vi "picoharp_close_device_handle.vi"(8 "error in (no error)":errorcluster, 11 "hydraharp in":refnum<class "picoharp.lvclass">) -> (0 "error out":errorcluster, 3 "hydraharp out":refnum<class "picoharp.lvclass">)   [LabVIEW 2015, in "picoharp.lvclass"]
uses:
  picoharp.lvclass
  picoharp.lvclass/picoharp.ctl
  phlib.dll
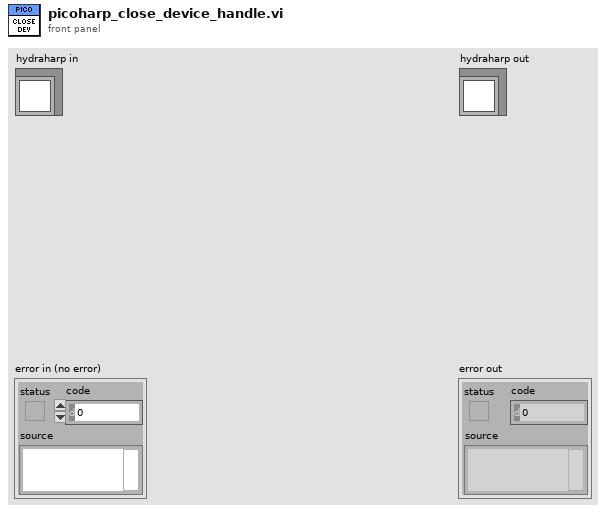
[diagram p1: front panel]
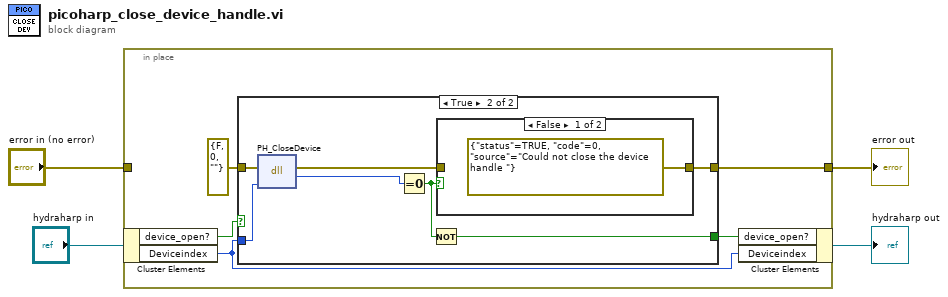
[diagram p0: block diagram]
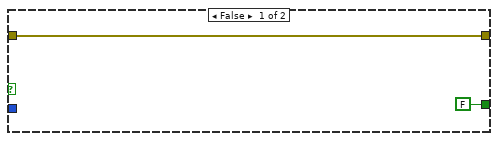
[diagram p2: hidden frame]
diagram:
  n1 = in-place {
    in-place-border: "error in (no error)" -> [_]
    in-place-border: [w7] -> w3
    n2 = in-place-cluster #1("hydraharp in") -> ("device_open?"=w9:bool, "Deviceindex"=w8:i32)
    n3 = case shown="True" w9 {
      tunnel: w8 -> [_ w18]
      tunnel: errorcluster {"status"=FALSE, "code"=0, "source"=""} ("error in (no error)") -> [w11 w17]
      tunnel: [w11 w13] -> w7
      tunnel: [FALSE w16] -> w6
      frame False {
      }
      frame True {
        n4 = dll-call lib="phlib.dll" fn="PH_CloseDevice"(error in=w17, "devidx"=w18) -> (error out=w14:errorcluster, "return type"=w12:i32)  [unwired: 3 in, 1 out]
        n5 = Equal To 0?(x=w12) -> (x = 0?=w15:bool)
        n6 = Not(x=w15) -> (.not. x?=w16:bool)
        n7 = case shown="False" w15 {
          tunnel: w14 -> [_ w20]
          tunnel: [errorcluster {"status"=TRUE, "code"=0, "source"="Could not close the device handle "} ("error out") w20] -> w13
          frame False {
          }
          frame True {
          }
        }
      }
    }
    n8 = in-place-cluster #1("device_open?"=w6, "Deviceindex"=w8) -> (→"hydraharp out":refnum<class "picoharp.lvclass">)
  }
  "error out" <- w3
